vi "Get LV EXE Path.vi"(10 "LabVIEW Version Number":dbl) -> (2 "appended path":path)   [LabVIEW 2013]
doc: "Takes the LabVIEW version number and builds the path to the LabVIEW.exe program (e.g. 9.0 to LabVIEW 2009)"
uses:
  <vilib>/Utility/sysdir.llb/System Directory Type.ctl
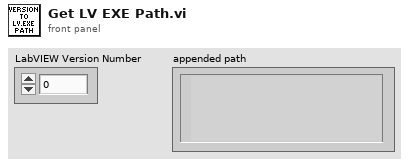
[diagram p1: front panel]
types:
  T1 = typedef "System Directory Type.ctl" = i32
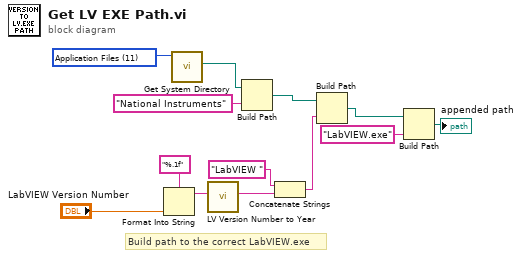
[diagram p0: block diagram]
diagram:
  w6 = T1 11 items=["User Home"=0, "User Desktop"=1, "User Documents"=2, "User Application Data"=3, "User Preferences"=4, "User Temporary"=5, "Public Documents"=6, "Public Application Data"=7, "Public Preferences"=8, "Public Cache"=13, "System Core Libraries"=9, "System Installed Libraries"=10, "Application Files"=11, "Boot Volume Root"=12] ("system directory type")
  # "Build path to the correct LabVIEW.exe"
  n1 = Format Into String(format string="%.1f", "LabVIEW Version Number") -> (resulting string=w3:string)  [unwired: 2 in, 1 out]
  n2 = call <vilib>:"Get System Directory.vi"("system directory type"=w6) -> ("system directory"=w7:path)  [unwired: 10 in]
  n3 = call "LV Version Number to Year.vi"("VI Version"=w3) -> ("LabVIEW Version"=w4:string)  [unwired: 10 in]
  n4 = Build Path(base path=w7, name or relative path="National Instruments") -> (appended path=w9:path)
  n5 = Concatenate Strings("LabVIEW " ("string"), w4) -> (w10:string)
  n6 = Build Path(base path=w9, name or relative path=w10) -> (appended path=w11:path)
  n7 = Build Path(base path=w11, name or relative path="LabVIEW.exe") -> (appended path=→"appended path":path)
